vi "FFT 1D single 2 cplx.vi"(5 "Normalize (True)":bool=TRUE, 7 "return only positive frequencies (True)":bool=TRUE, 8 "error in (no error)":errorcluster, 11 "y":sgl[](array[numeric])) -> (0 "error out":errorcluster, 1 "arg(Y) [rad]":sgl[](array[numeric]), 2 "amp(Y)":sgl[](array[numeric]), 3 "Y":csg[](array[numeric]))   [LabVIEW 2020, in "FFTWDLL.lvlib"]
doc: "Top level 1D FFT with single real input. Combines all FFTW steps (allocations, planing, freeing memory). May not be effective for repeated calls!"
uses:
  FFTWDLL.lvlib
  fftw_const_flags.ctl
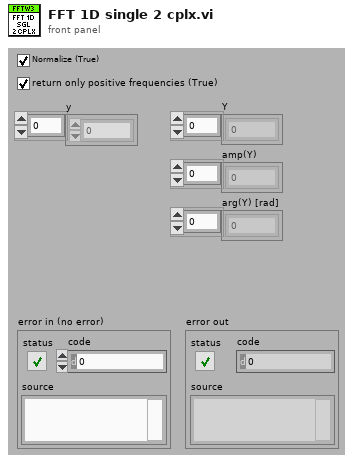
[diagram p1: front panel]
types:
  T1 = typedef "FFTWDLL.lvlib/fftw_const_flags.ctl" = cluster{"FFTW_MEASURE":bool, "FFTW_DESTROY_INPUT":bool, "FFTW_UNALIGNED":bool, "FFTW_CONSERVE_MEMORY":bool, "FFTW_EXHAUSTIVE":bool, "FFTW_PRESERVE_INPUT":bool, "FFTW_PATIENT":bool, "FFTW_ESTIMATE":bool, "FFTW_ESTIMATE_PATIENT":bool, "FFTW_BELIEVE_PCOST":bool, "FFTW_NO_DFT_R2HC":bool, "FFTW_NO_NOTHREAD":bool, "FFTW_NO_BUFFERING":bool, "FFTW_NO_INDIRECT_OP":bool, "FFTW_ALLOW_LARGE_GENERIC":bool, "FFTW_NO_RANK_SPLITS":bool, "FFTW_NO_VRANK_SPLITS":bool, "FFTW_NO_VRESCUE":bool, "FFTW_NO_SIMD":bool, "FFTW_NO_SLOW":bool, "FFTW_NO_FIXED_RADIX_LARGE_N":bool, "FFTW_ALLOW_PRUNING":bool, "FFTW_WISDOM_ONLY":bool}
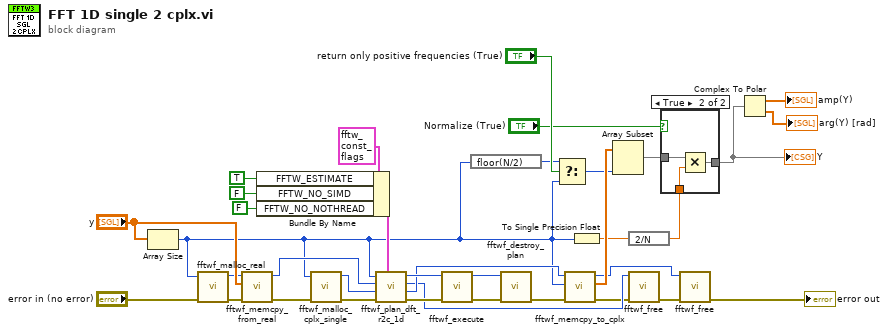
[diagram p0: block diagram]
diagram:
  n1 = Array Size(array="y") -> (size(s)=w4:i32)
  n2 = call "fftwf_malloc_real.vi"("error in (no error)"="error in (no error)", "single count"=w4) -> ("error out"=w31:errorcluster, "*data"=w29:u64)  [unwired: 8 in]
  n3 = call "fftwf_memcpy_from_real.vi"("error in (no error)"=w31, "source dbl array"="y", "*data_out"=w29) -> ("error out"=w26:errorcluster, "*data_out (copy)"=w28:u64)  [unwired: 7 in]
  n4 = Bundle By Name(cluster=T1 {"FFTW_MEASURE"=FALSE, "FFTW_DESTROY_INPUT"=FALSE, "FFTW_UNALIGNED"=FALSE, "FFTW_CONSERVE_MEMORY"=FALSE, "FFTW_EXHAUSTIVE"=FALSE, "FFTW_PRESERVE_INPUT"=FALSE, "FFTW_PATIENT"=FALSE, "FFTW_ESTIMATE"=FALSE, "FFTW_ESTIMATE_PATIENT"=FALSE, "FFTW_BELIEVE_PCOST"=FALSE, "FFTW_NO_DFT_R2HC"=FALSE, "FFTW_NO_NOTHREAD"=FALSE, "FFTW_NO_BUFFERING"=FALSE, "FFTW_NO_INDIRECT_OP"=FALSE, "FFTW_ALLOW_LARGE_GENERIC"=FALSE, "FFTW_NO_RANK_SPLITS"=FALSE, "FFTW_NO_VRANK_SPLITS"=FALSE, "FFTW_NO_VRESCUE"=FALSE, "FFTW_NO_SIMD"=FALSE, "FFTW_NO_SLOW"=FALSE, "FFTW_NO_FIXED_RADIX_LARGE_N"=FALSE, "FFTW_ALLOW_PRUNING"=FALSE, "FFTW_WISDOM_ONLY"=FALSE} ("FFTW flags"), "FFTW_ESTIMATE"=TRUE, "FFTW_NO_SIMD"=FALSE, "FFTW_NO_NOTHREAD"=FALSE) -> (w34:T1)
  n5 = call "fftwf_malloc_cplx_single.vi"("error in (no error)"=w26, "cplx double count"=w4) -> ("error out"=w35:errorcluster, "*data"=w27:u64)  [unwired: 8 in]
  n6 = call "fftwf_plan_dft_r2c_1d.vi"("FFTW flags"=w34, "error in (no error)"=w35, "*output_data"=w27, "*input_data"=w28, "N"=w4) -> ("error out"=w25:errorcluster, "*output_data (copy)"=w23:u64, "*input_data (copy)"=w19:u64, "*plan"=w24:u64)  [unwired: 3 in]
  n7 = call "fftwf_execute.vi"("error in (no error)"=w25, "*plan"=w24) -> ("error out"=w22:errorcluster, "*plan (copy)"=w20:u64)  [unwired: 8 in]
  n8 = expression code="floor(N/2)"(w4) -> (w17:i32)
  n9 = call "fftwf_destroy_plan.vi"("error in (no error)"=w22, "*plan"=w20) -> ("error out"=w21:errorcluster)  [unwired: 9 in]
  n10 = Select(t=w17, s="return only positive frequencies (True)", f=w4) -> (s? t:f=w15:i32)
  n11 = call "fftwf_memcpy_to_cplx.vi"("error in (no error)"=w21, "cplx count"=w4, "*data_in"=w23) -> ("error out"=w11:errorcluster, "cplx sgl array out"=w16:csg[], "*data_in (copy)"=w9:u64)  [unwired: 6 in]
  n12 = To Single Precision Float(number=w4) -> (single precision float=w2:sgl)
  n13 = Array Subset(array=w16, length=w15) -> (w6:csg[])  [unwired: 1 in]
  n14 = expression code="2/N"(w2) -> (w3:sgl)
  n15 = call "fftwf_free.vi"("error in (no error)"=w11, "*data"=w19) -> ("error out"=w12:errorcluster)  [unwired: 9 in]
  n16 = case shown="True" "Normalize (True)" {
    tunnel: w6 -> [w37 w40]
    tunnel: [w37 w39] -> w5
    tunnel: w3 -> [_ w38]
    frame False {
    }
    frame True {
      n17 = Multiply(x=w40, y=w38) -> (x*y=w39:csg[])
    }
  }
  "Y" <- w5
  n18 = call "fftwf_free.vi"("error in (no error)"=w12, "*data"=w9) -> ("error out"=→"error out":errorcluster)  [unwired: 9 in]
  n19 = Complex To Polar(r * e^(i*theta)=w5) -> (r=→"amp(Y)":sgl[], theta=→"arg(Y) [rad]":sgl[])
